vi "Teleop.vi"(10 "Match Info":T1={"Autonomous Elapsed Seconds"=0.0, "TeleOp Elapsed Seconds"=0.0, "Disabled Elapsed Seconds"=0.0, "Visited Autonomous"=FALSE, "Visited TeleOp"=FALSE, "Visited Disabled"=FALSE, "Autonomous Settings"={"Autonomous Style"=enum."Independent", "VI Refnum"=refnum}}, 11 "Call Context":T2) -> ()   [LabVIEW 2017]
doc: "This VI is called for each TeleOp packet received from the DS where the robot is not disabled. It is often used to read from the joysticks and update I/O or to update setpoints for timed control loops. It should complete and return within 20 milliseconds or it may miss DS packets."
uses:
  <vilib>/Rock Robotics/WPI/DriverStation/WPI_DriverStationDerivedRobotMode.ctl
  <vilib>/Rock Robotics/WPI/DriverStation/WPI_DriverStationMatch Info.ctl
  <vilib>/Rock Robotics/Network Tables/NT Read Boolean.vi
  <vilib>/Rock Robotics/Network Tables/NT Read Number.vi
  <vilib>/Rock Robotics/WPI/Utilities/WPI_GetSetVariantRefNum.vi
  <vilib>/Rock Robotics/WPI/RobotDrive/WPI_RobotDriveArcadeDrive_Standard(NoSaturation).vi
panel:
  out "Sample Slider 0":dbl(slide) scale=0.0..5.0
  out "Sample Boolean 1":bool
  out "Sample Boolean 0":bool
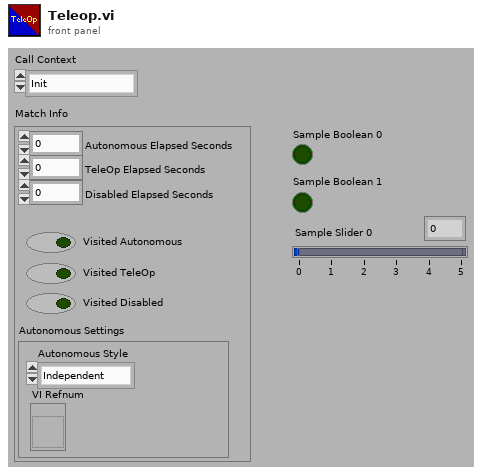
[diagram p1: front panel]
types:
  T1 = typedef "WPI_DriverStationMatch Info.ctl" = cluster{"Autonomous Elapsed Seconds":dbl, "TeleOp Elapsed Seconds":dbl, "Disabled Elapsed Seconds":dbl, "Visited Autonomous":bool, "Visited TeleOp":bool, "Visited Disabled":bool, "Autonomous Settings":cluster{"Autonomous Style":enum16{"Iterative", "Independent"}, "VI Refnum":refnum<vi>}}
  T2 = typedef "WPI_DriverStationDerivedRobotMode.ctl" = enum16{"Init", "Execute", "Stop"}
  T3 = typedef "WPI_JoystickDevRef.ctl" = cluster{"Device":T4}
  T4 = typedef "WPI_JoystickDeviceEnum.ctl" = enum16{"USB 0", "USB 1", "USB 2", "USB 3", "USB 4", "USB 5"}
  T5 = typedef "WPI_RobotDriveDevRef.ctl" = cluster{"DevStatus":errorcluster, "Motors[]":T6[], "Square Inputs":bool, "Max Output":dbl}
  T6 = typedef "WPI_MotorControlDeviceRef.ctl" = cluster{"DeviceStatus":errorcluster, "Type":T7, "PWM":cluster{"PWM Channel":T8, "DeadBand":T9}, "CAN":cluster{"Device Number":u8, "SetOutput VI Ref":variant, "GetOutput VI Ref":variant, "Enable VI Ref":variant, "Disable VI Ref":variant, "Data":variant}, "Invert":bool, "DIO PWM":cluster{"PWM \"Enable\" Channel":T8, "DIOChannel":T10, "PWM Rate":dbl}}
  T7 = typedef "WPI_MotorControlType.ctl" = enum16{"PWM", "CAN", "DIO PWM"}
  T8 = typedef "FPGA_DIOPWMChannel.ctl" = enum8{"PWM 0", "PWM 1", "PWM 2", "PWM 3", "PWM 4", "PWM 5", "PWM 6", "PWM 7", "PWM 8", "PWM 9", "PWM MXP 0", "PWM MXP 1", "PWM MXP 2", "PWM MXP 3", "PWM MXP 4", "PWM MXP 5", "PWM MXP 6", "PWM MXP 7", "PWM MXP 8", "PWM MXP 9", "Invalid"}
  T9 = typedef "WPI_PWMDeadband.ctl" = cluster{"Name":string, "maxPositivePwm":i32, "minPositivePwm":i32, "centerPwm":i32, "maxNegativePwm":i32, "minNegativePwm":i32, "angularRange":u16}
  T10 = typedef "FPGA_DIOChannel.ctl" = enum8{"DIO 0", "DIO 1", "DIO 2", "DIO 3", "DIO 4", "DIO 5", "DIO 6", "DIO 7", "DIO 8", "DIO 9", "DIO MXP 0", "DIO MXP 1", "DIO MXP 2", "DIO MXP 3", "DIO MXP 4", "DIO MXP 5", "DIO MXP 6", "DIO MXP 7", "DIO MXP 8", "DIO MXP 9", "DIO MXP 10", "DIO MXP 11", "DIO MXP 12", "DIO MXP 13", "DIO MXP 14", "DIO MXP 15", "SPI Port CS1", "SPI Port CS2", "SPI Port CS3", "SPI Port MISO", "SPI Port MOSI", "Invalid"}
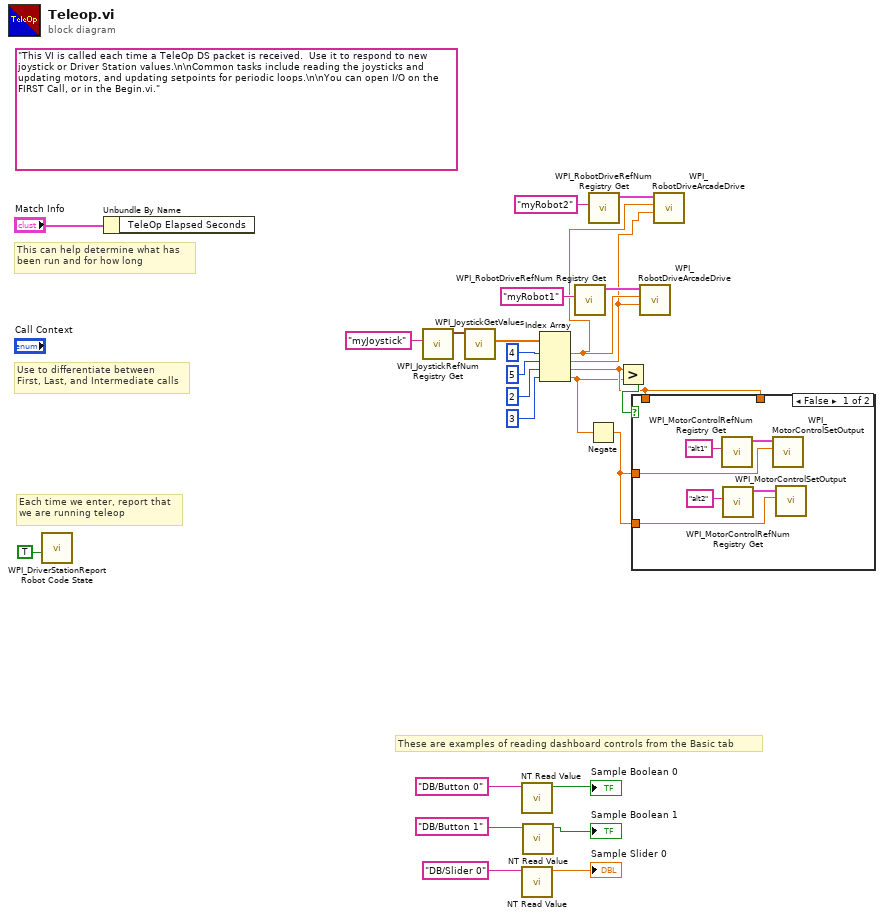
[diagram p0: block diagram]
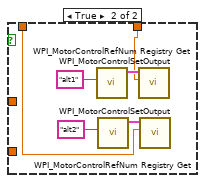
[diagram p2: hidden frame]
diagram:
  (unwired) "This VI is called each time a TeleOp DS packet is received.  Use it to respond to new joystick or Driver Station values.\n\nCommon tasks include reading the joysticks and updating motors, and updating setpoints for periodic loops.\n\nYou can open I/O on the FIRST Call, or in the Begin.vi."
  # "These are examples of reading dashboard controls from the Basic tab"
  # "Each time we enter, report that\nwe are running teleop"
  # "Use to differentiate between\nFirst, Last, and Intermediate calls"
  # "This can help determine what has\nbeen run and for how long"
  n1 = call <vilib>:"WPI_DriverStationReport Robot Code State.vi"("TeleOp"=TRUE ("Autonomous")) -> ()  [unwired: 10 in, 1 out]
  n2 = Unbundle By Name("Match Info") -> ()  [unwired: 1 out]
  n3 = call <vilib>:"WPI_JoystickRefNum Registry Get.vi"("refnum name"="myJoystick") -> ("JoystickDevRef"=w14:T3)  [unwired: 9 in, 1 out]
  n4 = call <vilib>:"WPI_JoystickGetValues.vi"("JoystickDevRef"=w14) -> ("Axes"=w13:dbl[])  [unwired: 6 in, 4 out]
  n5 = call-poly <vilib>:"NT Read Value.vi"("Name"="DB/Button 0" ("refnum name")) -> ("Boolean"=→"Sample Boolean 0":bool)  [unwired: 9 in, 1 out]
  n6 = call-poly <vilib>:"NT Read Value.vi"("Name"="DB/Slider 0" ("refnum name")) -> ("Numeric"=→"Sample Slider 0":dbl)  [unwired: 9 in, 1 out]
  n7 = call-poly <vilib>:"NT Read Value.vi"("Name"="DB/Button 1" ("refnum name")) -> ("Boolean"=→"Sample Boolean 1":bool)  [unwired: 9 in, 1 out]
  n8 = Index Array(array=w13, index #1=4 ("index"), index #2=5 ("index"), index #3=2 ("index"), index #4=3 ("index")) -> (element #1=w2:dbl, element #2=w1:dbl, element #3=w7:dbl, element #4=w5:dbl)
  n9 = call <vilib>:"WPI_RobotDriveRefNum Registry Get.vi"("refnum name"="myRobot1") -> ("RobotDriveDevRef"=w16:T5)  [unwired: 9 in, 1 out]
  n10 = Negate(x=w5) -> (-x=w6:dbl)
  n11 = call <vilib>:"WPI_RobotDriveRefNum Registry Get.vi"("refnum name"="myRobot2") -> ("RobotDriveDevRef"=w3:T5)  [unwired: 9 in, 1 out]
  n12 = Greater?(x=w7, y=w5) -> (0:w8:bool)
  n13 = case shown="False" w8 {
    tunnel: w7 -> [_ w33]
    tunnel: w7 -> [_ w32]
    tunnel: w6 -> [w27 _]
    tunnel: w6 -> [w26 _]
    frame False {
      n14 = call <vilib>:"WPI_MotorControlRefNum Registry Get.vi"("refnum name"="alt1") -> ("MotorControlDevRef"=w29:T6)  [unwired: 9 in, 1 out]
      n15 = call <vilib>:"WPI_MotorControlRefNum Registry Get.vi"("refnum name"="alt2") -> ("MotorControlDevRef"=w28:T6)  [unwired: 9 in, 1 out]
      n16 = call <vilib>:"WPI_MotorControlSetOutput.vi"("Output"=w27, "MotorControlDevRef"=w29) -> ()  [unwired: 7 in, 3 out]
      n17 = call <vilib>:"WPI_MotorControlSetOutput.vi"("Output"=w26, "MotorControlDevRef"=w28) -> ()  [unwired: 7 in, 3 out]
    }
    frame True {
      n18 = call <vilib>:"WPI_MotorControlRefNum Registry Get.vi"("refnum name"="alt1") -> ("MotorControlDevRef"=w35:T6)  [unwired: 9 in, 1 out]
      n19 = call <vilib>:"WPI_MotorControlRefNum Registry Get.vi"("refnum name"="alt2") -> ("MotorControlDevRef"=w34:T6)  [unwired: 9 in, 1 out]
      n20 = call <vilib>:"WPI_MotorControlSetOutput.vi"("Output"=w33, "MotorControlDevRef"=w35) -> ()  [unwired: 7 in, 3 out]
      n21 = call <vilib>:"WPI_MotorControlSetOutput.vi"("Output"=w32, "MotorControlDevRef"=w34) -> ()  [unwired: 7 in, 3 out]
    }
  }
  n22 = call-poly <vilib>:"WPI_RobotDriveArcadeDrive.vi"("Y axis value"=w1, "X axis value"=w2, "RobotDriveDevRef"=w16) -> ()  [unwired: 6 in, 3 out]
  n23 = call-poly <vilib>:"WPI_RobotDriveArcadeDrive.vi"("Y axis value"=w1, "X axis value"=w2, "RobotDriveDevRef"=w3) -> ()  [unwired: 6 in, 3 out]
